vi "splitByDevice.vi"(8 "error in (no error)":errorcluster, 10 "DeviceArray":refnum<class "DeviceArray.lvclass">, 11 "ScriptEventList in":refnum<class "ScriptEventList.lvclass">) -> (0 "error out":errorcluster, 2 "DeviceArray out":refnum<class "DeviceArray.lvclass">, 3 "ScriptEventList out":refnum<class "ScriptEventList.lvclass">)   [LabVIEW 2009, in "Tools.lvlib" / "Scripting.lvlib" / "ScriptEventList.lvclass"]
uses:
  ScriptEventList.lvclass
  DatabaseHelpers/Database Objects/DeviceArray/DeviceArray.lvclass
  ScriptEventList.lvclass/ScriptEventList.ctl
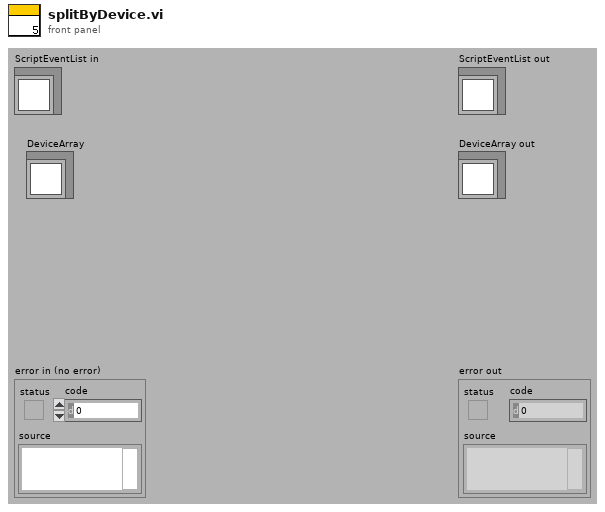
[diagram p1: front panel]
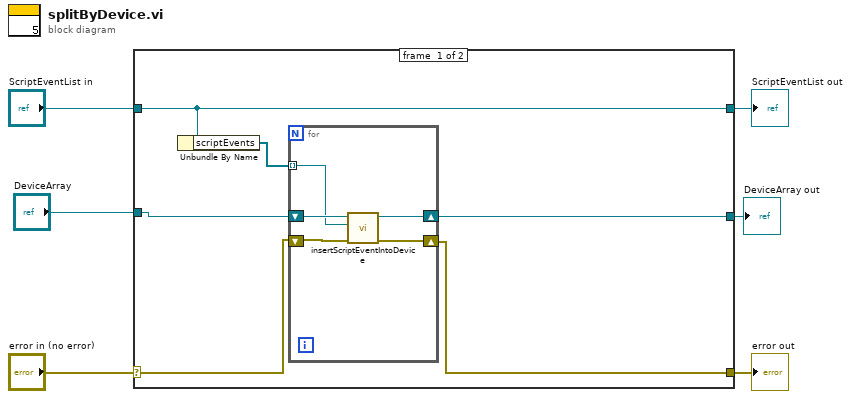
[diagram p0: block diagram]
diagram:
  n1 = case shown="No Error" "error in (no error)" {
    selector: "error in (no error)" -> [w9 w19]
    tunnel: [w8 w19] -> w5
    tunnel: [w12 w18] -> w3
    tunnel: "ScriptEventList in" -> [w12 w18]
    tunnel: "DeviceArray" -> [w10 _]
    tunnel: [w7 _] -> w1
    frame #0 {
      n2 = Unbundle By Name(w12) -> ("scriptEvents"=w11:refnum<class "ScriptEvent.lvclass">[])
      n3 = for {
        tunnel: w11 -> [w16] mode=indexing
        shift-right: [w14] -> w7
        shift-left: w10 -> [w17]
        shift-right: [w13] -> w8
        shift-left: w9 -> [w15]
        n4 = call "insertScriptEventIntoDevice.vi"("error in (no error)"=w15, "ScriptEvent"=w16, "DeviceArray in"=w17) -> ("error out"=w13:errorcluster, "DeviceArray out"=w14:refnum<class "DeviceArray.lvclass">)  [unwired: 7 in]
      }
    }
    frame #1 {
    }
  }
  "error out" <- w5
  "ScriptEventList out" <- w3
  "DeviceArray out" <- w1
